vi "ReadVISA.vi"(0 "object in":refnum<class "DAQ.lvclass">, 5 "error in (no error)":errorcluster) -> (14 "object out":refnum<class "DAQ.lvclass">, 16 "Scale Data":dbl, 19 "error out":errorcluster)   [LabVIEW 2021, in "DAQ.lvclass"]
uses:
  DAQ.lvclass
  DAQ.lvclass/DAQ.ctl
panel:
  in  "string to write 2":string="Q\r\n"
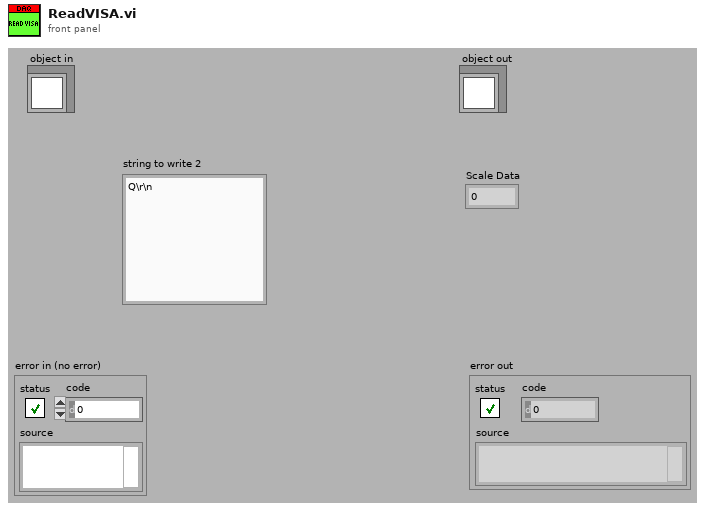
[diagram p1: front panel]
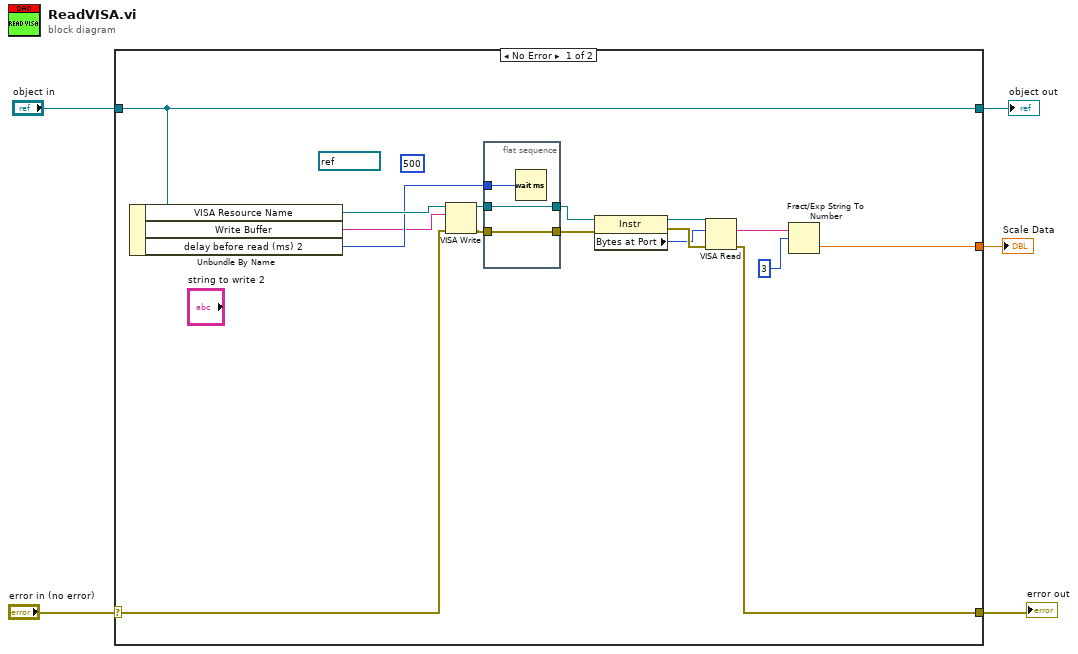
[diagram p0: block diagram]
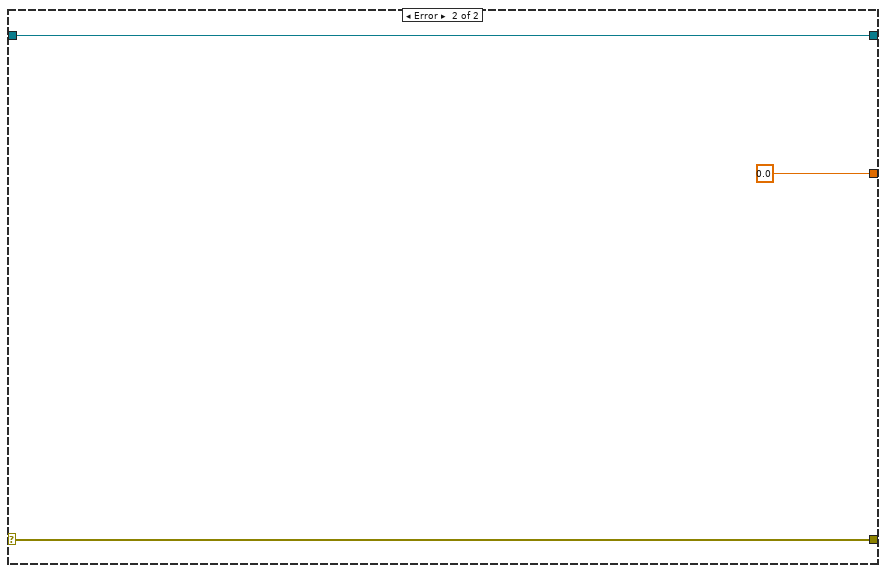
[diagram p2: hidden frame]
diagram:
  n1 = case shown="No Error" "error in (no error)" {
    selector: "error in (no error)" -> [w10 w27]
    tunnel: [w13 w27] -> w1
    tunnel: [w9 w26] -> w3
    tunnel: "object in" -> [w9 w26]
    tunnel: [w21 0.0] -> w2
    frame No Error {
      (unwired) u32 500 ("milliseconds to wait")
      (unwired) refnum<visa-resource-name> "COM7" ("VISA resource name")
      n2 = Unbundle By Name(w9) -> ("VISA Resource Name"=w8:refnum<visa-resource-name>, "Write Buffer"=w6:string, "delay before read (ms) 2"=w7:u32)
      n3 = VISA Write(VISA resource name=w8, write buffer=w6, error in (no error)=w10) -> (VISA resource name out=w18:refnum<visa-resource-name>, error out=w19:errorcluster)  [unwired: 1 out]
      n4 = flat-sequence {
        tunnel: [w24] -> w20
        tunnel: w19 -> [w24]
        tunnel: w18 -> [w23]
        tunnel: [w23] -> w17
        tunnel: w7 -> [w22]
        frame #0 {
          n5 = Wait (ms)(milliseconds to wait=w22) -> ()  [unwired: 1 out]
        }
      }
      n6 = property on="Property Node" class="Instr"(reference=w17, error in=w20) -> (reference out=w16:refnum<visa-resource-name>, error out=w15:errorcluster, "Bytes at Port"=w14:u32)
      n7 = VISA Read(VISA resource name=w16, byte count=w14, error in (no error)=w15) -> (read buffer=w12:string, error out=w13:errorcluster)  [unwired: 2 out]
      n8 = Fract/Exp String To Number(string=w12, offset=3) -> (number=w21:dbl)  [unwired: 2 in, 1 out]
    }
    frame Error {
    }
  }
  "error out" <- w1
  "object out" <- w3
  "Scale Data" <- w2
